vi "HEWH Remove Channel.vi"(11 "Agilent Channel Input in":string="111,112,113,114,115,116,109,110,201,202,203,204,205,206,207,208,209,210,211,212,213,214,215,216,107,108,301,302,303,304,305,306,307,308,309,310,311,312,313,314,315,316,105,106") -> (3 "Channel Removed":string)   [LabVIEW 2023]
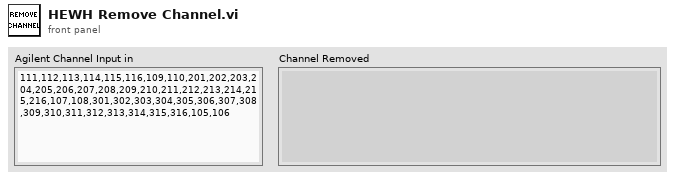
[diagram p1: front panel]
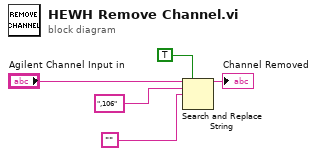
[diagram p0: block diagram]
diagram:
  n1 = Search and Replace String(replace all?=TRUE ("replace all? (F)"), input string="Agilent Channel Input in", search string=",106", replace string="") -> (result string=→"Channel Removed":string)  [unwired: 4 in, 3 out]
